vi "Logitech Webcam.vi"() -> ()   [LabVIEW 2011]
uses:
  _GlobalVariables&Libraries/ATV Program Global Variables.vi
  <vilib>/vision/NI_Vision_Development_Module.lvlib
panel:
  out "Left":sgl
  out "Bottom":sgl
  out "Right":sgl
  out "Top":sgl
  out "Turn Left":bool
  out "Turn Right":bool
  out "Stay Straight":bool
  out "Left 2":sgl
  out "Bottom 2":sgl
  out "Right 2":sgl
  out "Top 2":sgl
  out "Area Occupied to the Left":sgl
  out "Area Occupied to the Right":sgl
  in  "(Pixel^2)":sgl=300.0
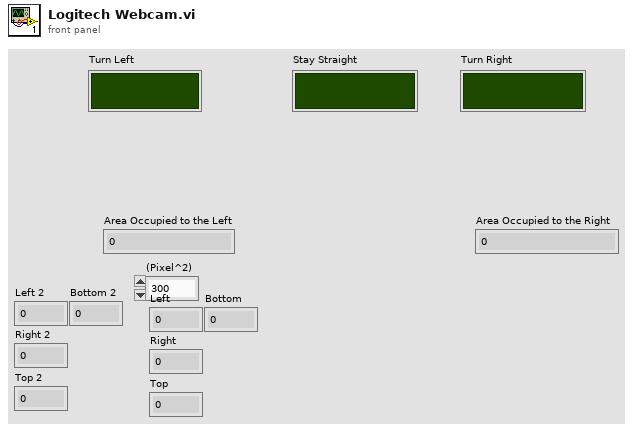
[diagram p1: front panel]
types:
  T1 = typedef "IMAQ Image.ctl" = refnum<image>
  T2 = cluster{"Clamp Settings":cluster{"Contrast":i32, "Filter width":i32, "Steepness":i32, "Subsampling Ratio":u32, "Show Search Area":bool, "Show Search Lines":bool, "Show Edges Found":bool, "Show Result":bool}, "Color Plane":i32, "BCG":cluster{"Brightness":sgl, "Contrast":sgl, "Gamma":sgl}}
  T3 = cluster{"End ATV Program":bool, "E-Stop":bool, "Save Logfile":bool, "Logfile Iteration Delay (ms)":u32, "Loop iteration time (ms)":u32, "Logfile Location":path, "Default GPS Navigation Path":path, "Computer":string, "Default GPS Boundary Path":path}
  T4 = cluster{"Brightness":sgl, "Contrast":sgl, "Gamma":sgl}
  T5 = cluster{"Contrast":i32, "Filter width":i32, "Steepness":i32, "Subsampling Ratio":u32, "Show Search Area":bool, "Show Search Lines":bool, "Show Edges Found":bool, "Show Result":bool}
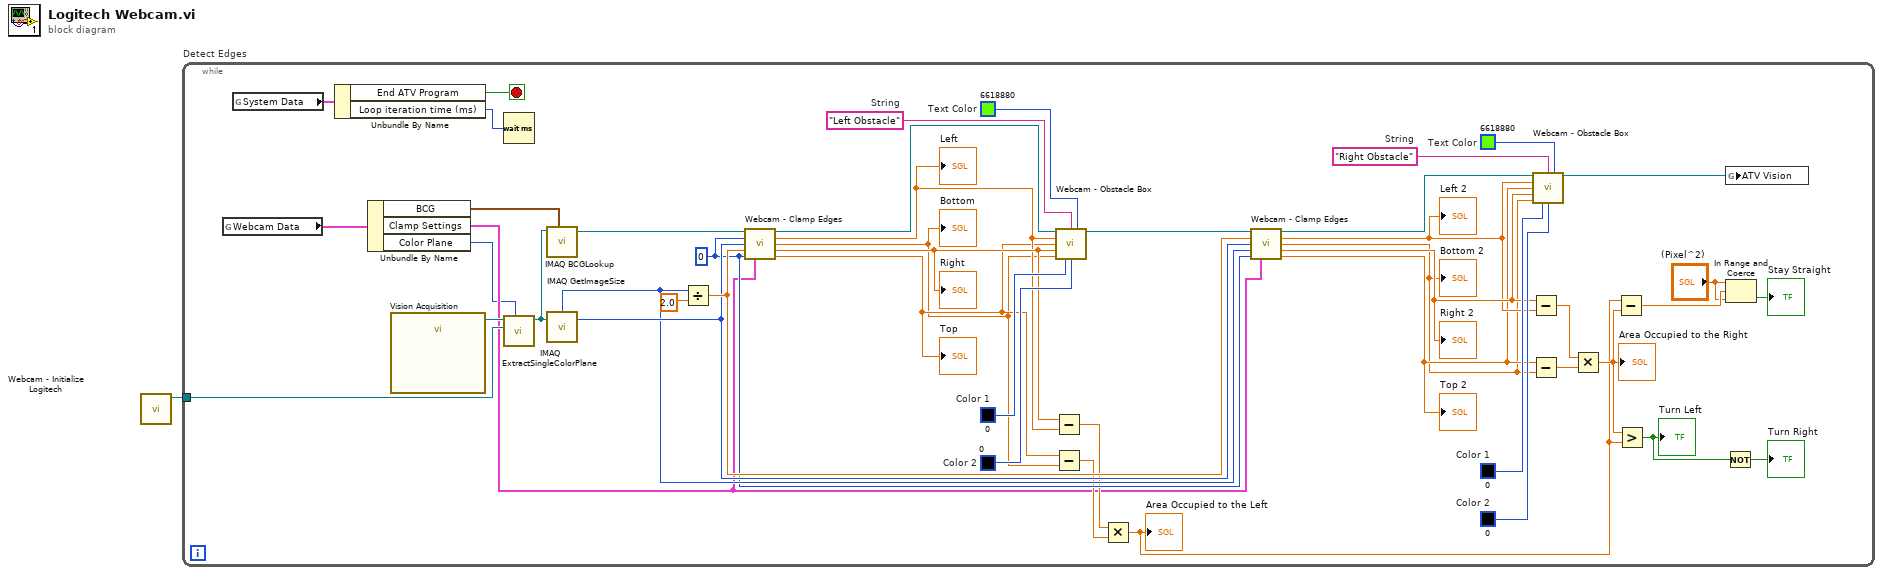
[diagram p0: block diagram]
diagram:
  n1 = call "Webcam - Initialize Logitech.vi"() -> ("New Image"=w1:T1)  [unwired: 10 in, 1 out]
  n2 = while "Detect Edges" {
    tunnel: w1 -> [w13]
    stop <- w9 stop-if-true
    w33 = 0 ("Search Area Left")
    w42 = u32 6618880  # Text Color
    w41 = "Right Obstacle"  # String
    w40 = u32 0  # Color 2
    w39 = u32 0  # Color 1
    w45 = u32 6618880  # Text Color
    w46 = "Left Obstacle"  # String
    w47 = u32 0  # Color 2
    w48 = u32 0  # Color 1
    n3 = global read "ATV Program Global Variables.vi" "Webcam Data"() -> (w8:T2)
    n4 = global read "ATV Program Global Variables.vi" "System Data"() -> (w11:T3)
    n5 = Unbundle By Name(w11) -> ("End ATV Program"=w9:bool, "Loop iteration time (ms)"=w10:u32)
    n6 = Unbundle By Name(w8) -> ("BCG"=w2:T4, "Clamp Settings"=w7:T5, "Color Plane"=w6:i32)
    n7 = call "Vision Acquisition"() -> ("Image Out"=w12:T1)  [unwired: 26 in, 1 out]
    n8 = Wait (ms)(milliseconds to wait=w10) -> ()  [unwired: 1 out]
    n9 = call "IMAQ ExtractSingleColorPlane"("Color Plane"=w6, "Image Dst"=w13, "Image Src"=w12) -> ("Image Dst Out"=w4:T1)  [unwired: 7 in, 1 out]
    n10 = call "IMAQ BCGLookup"("Image Src"=w4, "BCG Values"=w2) -> ("Image Dst Out"=w3:T1)  [unwired: 3 in, 3 out]
    n11 = call "IMAQ GetImageSize"("Image"=w4) -> ("Y Resolution"=w35:i32, "X Resolution"=w34:i32)  [unwired: 3 in, 1 out]
    n12 = Divide(x=w34, y=2.0) -> (x/y=w36:dbl)
    n13 = call "Webcam - Clamp Edges.vi"("Image In"=w3, "Search Area Left"=w33, "Search Area Top"=w35, "Search Area Right"=w36, "Search Area Bottom"=w33, "Settings"=w7) -> ("Image Out"=w44:T1, "Left"=w31:sgl, "Bottom"=w29:sgl, "Right"=w32:sgl, "Top"=w30:sgl)  [unwired: 5 in]
    "Left" <- w31
    "Bottom" <- w29
    "Right" <- w32
    "Top" <- w30
    n14 = Subtract(x=w32, y=w31) -> (x-y=w28:sgl)
    n15 = Subtract(x=w30, y=w29) -> (x-y=w27:sgl)
    n16 = call "Webcam - Obstacle Box.vi"("Image In"=w44, "String"=w46, "Text Color"=w45, "Left"=w31, "Top"=w30, "Right"=w32, "Bottom"=w29, "Color 1"=w48, "Color 2"=w47) -> ("Image Out"=w37:T1)  [unwired: 6 in]
    n17 = Multiply(x=w28, y=w27) -> (x*y=w16:sgl)
    "Area Occupied to the Left" <- w16
    n18 = call "Webcam - Clamp Edges.vi"("Image In"=w37, "Search Area Left"=w36, "Search Area Top"=w35, "Search Area Right"=w34, "Search Area Bottom"=w33, "Settings"=w7) -> ("Image Out"=w43:T1, "Left"=w23:sgl, "Bottom"=w21:sgl, "Right"=w24:sgl, "Top"=w22:sgl)  [unwired: 5 in]
    "Left 2" <- w23
    "Bottom 2" <- w21
    "Right 2" <- w24
    "Top 2" <- w22
    n19 = Subtract(x=w24, y=w23) -> (x-y=w25:sgl)
    n20 = Subtract(x=w22, y=w21) -> (x-y=w26:sgl)
    n21 = call "Webcam - Obstacle Box.vi"("Image In"=w43, "String"=w41, "Text Color"=w42, "Left"=w23, "Top"=w22, "Right"=w24, "Bottom"=w21, "Color 1"=w39, "Color 2"=w40) -> ("Image Out"=w5:T1)  [unwired: 6 in]
    n22 = Multiply(x=w25, y=w26) -> (x*y=w17:sgl)
    "Area Occupied to the Right" <- w17
    n23 = Subtract(x=w16, y=w17) -> (x-y=w19:sgl)
    n24 = Greater?(x=w17, y=w16) -> (0:w14:bool)
    "Turn Left" <- w14
    n25 = Not(x=w14) -> (.not. x?=→"Turn Right":bool)
    n26 = global write "ATV Program Global Variables.vi" "ATV Vision"(w5) -> ()
    n27 = In Range and Coerce(upper limit="(Pixel^2)", x=w19, lower limit="(Pixel^2)") -> (In Range?=→"Stay Straight":bool)  [unwired: 1 out]
  }
